vi "slam.vi"(7 "X":dbl[](array[numeric]), 8 "error in":errorcluster, 9 "measurements":dbl[][](array[numeric]), 10 "dX":dbl[](array[numeric]), 11 "P":dbl[][](array[numeric])) -> (0 "error out":errorcluster, 1 "measuredLandmarks":dbl[][](array[numeric]), 2 "Xodometry":dbl[](array[numeric]), 3 "Pout":dbl[][](array[numeric]), 5 "Xout":dbl[](array[numeric]))   [LabVIEW 2009]
uses:
  C:/Users/Timon/Documents/LabVIEW Data/SLAM.m
  C:/Users/Timon/Documents/LabVIEW Data/MathScriptVIs/MCStatic_151019524_ba4b9d4e69408f9a0d39e6e0b59a83bc.vi
  C:/Users/Timon/Documents/LabVIEW Data/addLandmark.m
  C:/Users/Timon/Documents/LabVIEW Data/associateToLandmark.m
  C:/Users/Timon/Documents/LabVIEW Data/assOrAddLandmark.m
  C:/Users/Timon/Documents/LabVIEW Data/dist.m
  C:/Users/Timon/Documents/LabVIEW Data/distance.m
  C:/Users/Timon/Documents/LabVIEW Data/findRangeBearing.m
  C:/Users/Timon/Documents/LabVIEW Data/shiftAngle.m
  C:/Users/Timon/Documents/LabVIEW Data/updateFromLandmarks.m
  C:/Users/Timon/Documents/LabVIEW Data/updateFromOdometry.m
  <vilib>/imath/engines/lvmath2/RunTimeEngine/ErrorHandling/NIMS_Finalize Error.vi
  <vilib>/imath/engines/lvmath2/RunTimeEngine/Parser/MC_Version.vi
  <vilib>/imath/engines/lvmath2/RunTimeEngine/Managers/WorkSpace/UID Generator.vi
  <vilib>/imath/engines/lvmath2/RunTimeEngine/NodeEndStatement/NIMS_NodeEndStatement_Output.vi
  <instcachedir>/0/NIMS_NodeEndStatement_Output_B70DDD75627E4997AAE11E9955EDAA25.lvgen/NIMS_NodeEndStatement_Output_B70DDD75627E4997AAE11E9955EDAA25_004.vi
  <instcachedir>/0/NIMS_NodeEndStatement_Output_B70DDD75627E4997AAE11E9955EDAA25.lvgen/NIMS_NodeEndStatement_Output_B70DDD75627E4997AAE11E9955EDAA25_003.vi
  <instcachedir>/0/NIMS_NodeEndStatement_Output_B70DDD75627E4997AAE11E9955EDAA25.lvgen/NIMS_NodeEndStatement_Output_B70DDD75627E4997AAE11E9955EDAA25_002.vi
  <vilib>/imath/engines/lvmath2/RunTimeEngine/Managers/SymbolTable/Clear UID.vi
  <vilib>/imath/engines/lvmath/Functions/Error Handling/MergeErrorsWrapper.vi
  <instcachedir>/0/MCStatic_151019524_ba4b9d4e69408f9a0d39e6e0b59a83bc_CF1AE7649DA14147A24F2D226153A6C1.lvgen/MCStatic_151019524_ba4b9d4e69408f9a0d39e6e0b59a83bc_CF1AE7649DA14147A24F2D226153A6C1_000.vi
  <vilib>/imath/engines/lvmath2/RunTimeEngine/Managers/SymbolTable/NIMS_WorkSpace.lvlib
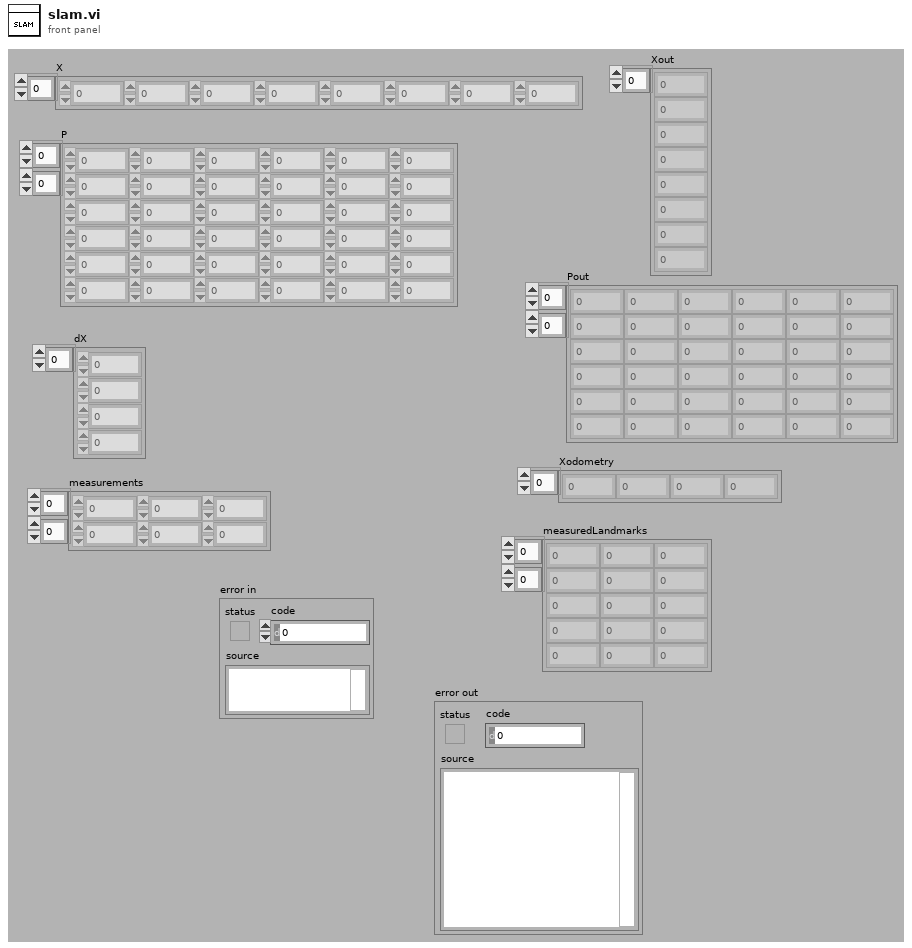
[diagram p1: front panel]
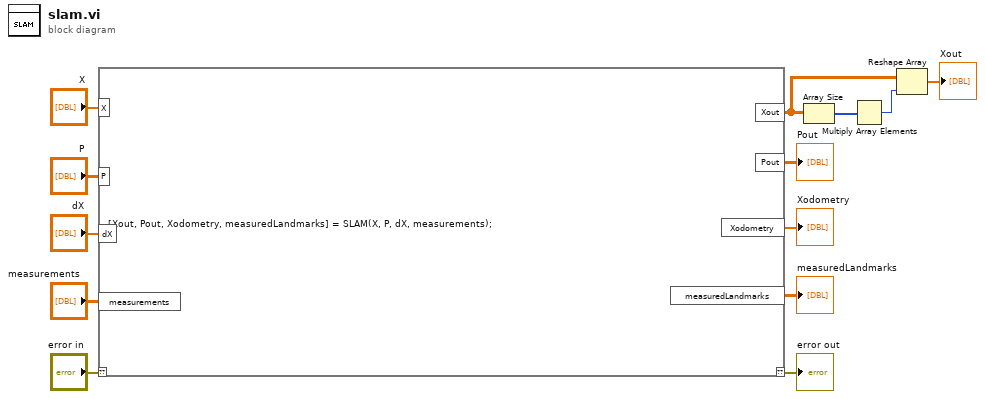
[diagram p0: block diagram]
diagram:
  n1 = mathscript code="[Xout, Pout, Xodometry, measuredLandmarks] = SLAM(X, P, dX, measurements);"("??"="error in", "X"="X", "P"="P", "dX"="dX", "measurements"="measurements") -> ("??"=→"error out":errorcluster, "Xout"=w2:cdb[][], "Pout"=→"Pout":cdb[][], "Xodometry"=→"Xodometry":dbl[], "measuredLandmarks"=→"measuredLandmarks":dbl[][])
  n2 = Array Size(array=w2) -> (size(s)=w4:i32[])
  n3 = Multiply Array Elements(1:w4) -> (0:w3:i32)
  n4 = Reshape Array(w2, w3) -> (→"Xout":cdb[])
